vi "ATM Main.vi"   [LabVIEW 2016, in "CLD Exam - ATM.lvlib"]
uses:
  CLD Exam - ATM.lvlib
  <vilib>/Utility/sysdir.llb/System Directory Type.ctl
  Error/Classes/Error Interface/Dialog Types.ctl
  Classes/Assembler/Assembler.lvclass
  Error/Stream Error.lvlib
  Error/Classes/Error Interface/Error Interface.lvclass
types:
  T1 = typedef "Stream Error.lvlib/Error Interface.lvclass/Dialog Types.ctl" = enum16{"No Dialog", "Continue Dialog", "Stop Dialog", "Abort Dialog"}
  T2 = typedef "System Directory Type.ctl" = i32
  T3 = enum32{"invalid app kind", "Development System", "Run Time System", "Student Edition", "Embedded LabVIEW", "Evaluation", "Custom"}
  T4 = enum32{"Invalid", "Standard", "Closed", "Hidden", "Minimized", "Maximized"}
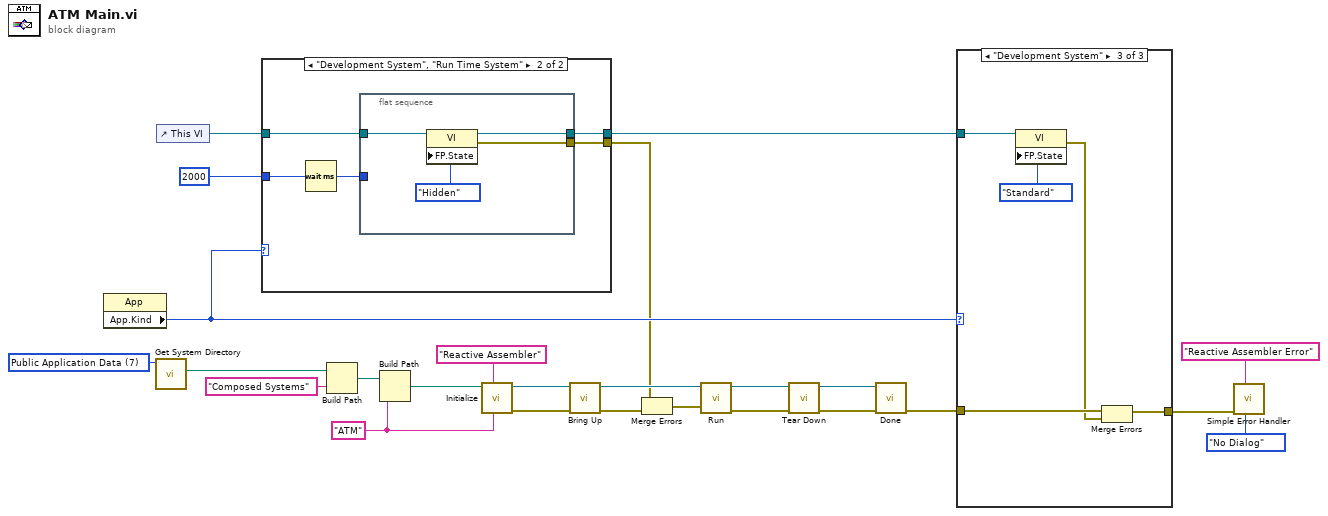
[diagram p0: block diagram]
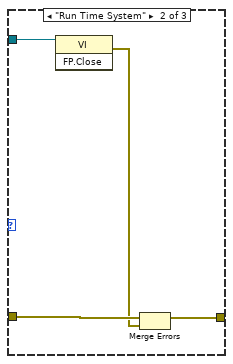
[diagram p3: hidden frame]
diagram:
  w23 = T2 7 items=["User Home"=0, "User Desktop"=1, "User Documents"=2, "User Application Data"=3, "User Preferences"=4, "User Temporary"=5, "Public Documents"=6, "Public Application Data"=7, "Public Preferences"=8, "Public Cache"=13, "System Core Libraries"=9, "System Installed Libraries"=10, "Application Files"=11, "Boot Volume Root"=12] ("system directory type")
  w21 = "ATM" ("iName")
  n1 = property class="App"() -> ("App.Kind"=w17:T3)  [unwired: 2 in, 2 out]
  n2 = call <vilib>:"Get System Directory.vi"("system directory type"=w23) -> ("system directory"=w22:path)  [unwired: 10 in]
  n3 = control-ref of="This VI"() -> (w18:refnum<vi>)
  n4 = case shown="\"Development System\", \"Run Time System\"" w17 {
    tunnel: u32 2000 ("milliseconds to wait") -> [_ w31]
    tunnel: w18 -> [w26 w29]
    tunnel: [w26 w28] -> w16
    tunnel: [_ w27] -> w9
    frame Default {
    }
    frame "Development System", "Run Time System" {
      n5 = Wait (ms)(milliseconds to wait=w31) -> (millisecond timer value=w30:u32)
      n6 = flat-sequence {
        tunnel: w30 -> [_]
        tunnel: w29 -> [w35]
        tunnel: [w34] -> w28
        tunnel: [w33] -> w27
        frame #0 {
          n7 = property class="VI"(reference=w35, "FP.State"=T4."Hidden" ("Front Panel Window:State")) -> (reference out=w34:refnum<vi>, error out=w33:errorcluster)  [unwired: 1 in]
        }
      }
    }
  }
  n8 = Build Path(base path=w22, name or relative path="Composed Systems") -> (appended path=w24:path)
  n9 = Build Path(base path=w24, name or relative path=w21) -> (appended path=w1:path)
  n10 = call "Initialize.vi"("iName"=w21, "iType"="Reactive Assembler", "Application Data"=w1) -> ("error out"=w8:errorcluster, "Assembler out"=w15:refnum<class "Assembler.lvclass">)  [unwired: 7 in]
  n11 = call "Bring Up.vi"("error in (no error)"=w8, "Assembler in"=w15) -> ("error out"=w10:errorcluster, "Assembler out"=w14:refnum<class "Assembler.lvclass">)  [unwired: 8 in]
  n12 = Merge Errors(w9, w10) -> (w11:errorcluster)
  n13 = call "Run.vi"("error in (no error)"=w11, "Assembler in"=w14) -> ("error out"=w7:errorcluster, "Assembler out"=w13:refnum<class "Assembler.lvclass">)  [unwired: 8 in]
  n14 = call "Tear Down.vi"("error in (no error)"=w7, "Assembler in"=w13) -> ("error out"=w6:errorcluster, "Assembler out"=w12:refnum<class "Assembler.lvclass">)  [unwired: 8 in]
  n15 = call "Done.vi"("error in (no error)"=w6, "Assembler in"=w12) -> ("error out"=w5:errorcluster)  [unwired: 9 in]
  n16 = case shown="\"Development System\"" w17 {
    tunnel: w16 -> [_ w40 w45]
    tunnel: w5 -> [w36 w39 w44]
    tunnel: [w36 w37 w42] -> w4
    frame Default {
    }
    frame "Run Time System" {
      n17 = invoke class="VI" method="FP.Close"(reference=w40) -> (error out=w38:errorcluster)  [unwired: 2 in, 2 out]
      n18 = Merge Errors(w39, w38) -> (w37:errorcluster)
    }
    frame "Development System" {
      n19 = property class="VI"(reference=w45, "FP.State"=T4."Standard" ("Front Panel Window:State")) -> (error out=w43:errorcluster)  [unwired: 1 in, 1 out]
      n20 = Merge Errors(w44, w43) -> (w42:errorcluster)
    }
  }
  n21 = call "Simple Error Handler.vi"("Dialog Type"=Dialog_Types."No Dialog", "Window Title"="Reactive Assembler Error", "Error In"=w4) -> ()  [unwired: 7 in, 2 out]
